vi "Nuevo Asistente.vi"(8 "error in (no error)":errorcluster) -> (0 "error out":errorcluster, 1 "Datos de Nueva Adquisición":T1={"Equipo a Utilizar"=enum."TDS 2012B Osciloscope", "Montura"=enum."Motor Bipolar", "Datos Zaber"={"Sentido de Adquisición"=FALSE, "Comenzar Desde Home?"=FALSE, "Distancia a recorrer (um)"=0.0, "Pasos motor"=0, "Distancia entre Lecturas (um)"=0.0, "Puerto"=""}, "Datos Bipolar/Unipolar"={"Puerto COM"="", "Pasos entre Lecturas"=0, "Numero de lecturas"=0, "Sentido del motor"=TRUE}, "Datos Archivo"={"Ruta Archivo"=path "", "Nombre de Prueba"=""}, "Datos actuales"={"Montura"="", "Equipo"="", "Posición Actual"="", "Distancia Total a recorrer"="", "distancia Entre lecturas"="", "Pasos entre lecturas"=""}, "Datos a Guardar In"={"Datos Cursor Tektronix"="", "Datos Lokin"="", "Posición Cero"=0.0, "Posición Actual"=0.0}, "Datos Osciloscopio"={"Sesión Visa Osciloscopio"="Tektronix_TDS2012C", "Tipo de Adquisición"=enum."Voltaje Pico Pico", "Canal a Utilizar"=enum."Canal 1", "Parametros de Adquisición"=enum."Una Muestra", "Número Promedio"=2}, "Datos Lock In"={"Visa Lock in"="Tektronix_TDS2012C"}} {"Datos Osciloscopio"."Número Promedio" min=2 max=20; "Datos a Guardar In"."Posición Actual" format="%#_10f"; "Datos a Guardar In"."Posición Cero" format="%#_10f"; "Datos Bipolar/Unipolar"."Numero de lecturas" max=910098 step=1}, 2 "Iniciar Prueba":bool)   [LabVIEW 2020]
doc: "Este VI es un asistente tipo \"wizzard\" para obtener los parámetros de una nueva prueba, captura el tipo de montura, cuantos pasos por lectura, equipo para lectura y ruta de almacenamiento de datos, nombre de la prueba."
uses:
  Type Definitions/tab wizard.ctl
  Type Definitions/Asistente de adquisicion Cluster.ctl
  Type Definitions/Datos a Guardar.ctl
  Type Definitions/datos osciloscopio.ctl
  Type Definitions/Datos Zaber.ctl
  Type Definitions/parametros motores.ctl
  <vilib>/Utility/sysdir.llb/System Directory Type.ctl
  H:/Mi unidad/Departamento de Ingenieria/Investigadores/Gabriel Ramos/Proyecto Monturas v13/LV Source/Type Definitions/Tipos de montura.ctl
panel:
  in  "Cancel Button":bool
  in  "Previous Button":bool
  in  "Next Button":bool
  out "Tab general":T7
  in  "Tipo de montura/Motor":T2
  in  "Datos Zaber":T3={"Sentido de Adquisición"=TRUE, "Comenzar Desde Home?"=TRUE, "Distancia a recorrer (um)"=2.0, "Pasos motor"=0, "Distancia entre Lecturas (um)"=0.1, "Puerto"="COM4"}
  in  "Datos Bipolar/Unipolar":T4 {"Numero de lecturas" max=910098 step=1}
  in  "Seleccion Equipo de medición":enum16{"SR830 Lock In", "TDS 2012B Osciloscope"}(ring)=enum."TDS 2012B Osciloscope"
  in  "Datos Osciloscopio":T6={"Sesión Visa Osciloscopio"="USB0::0x0699::0x0368::C017587::INSTR", "Tipo de Adquisición"=enum."Voltaje Pico Pico", "Canal a Utilizar"=enum."Canal 1", "Parametros de Adquisición"=enum."Una Muestra", "Número Promedio"=2} {"Número Promedio" min=2 max=20}
  in  "Puerto GPIB Lock In":refnum<visa-resource-name>="GPIB0::8::INSTR"
  in  "Datos Archivo":T8
  # "ENA"
  # "Bienvenido al Asistente de adquisición Automatizado\n\nEste asistente le ayudará a:\n\n* Seleccionar motor-montura a usar\n     -Zaber                  (USB-RS232C)\n     -Motor Unipolar     (COM Port)\n     -Motor Bipolar       (COM Port)\n\n* Seleccionar Instrumento de adquisición\n     -Lock-In Amplifier         SR830\n     -Osciloscopio               TDS-2012B\n\n* Parametros de adquisición\n    -Guardado de Archivo\n    -Pasos por lectura"
  # "Motor Unipolar"
  # "Motor Bipolar"
  # "Zaber"
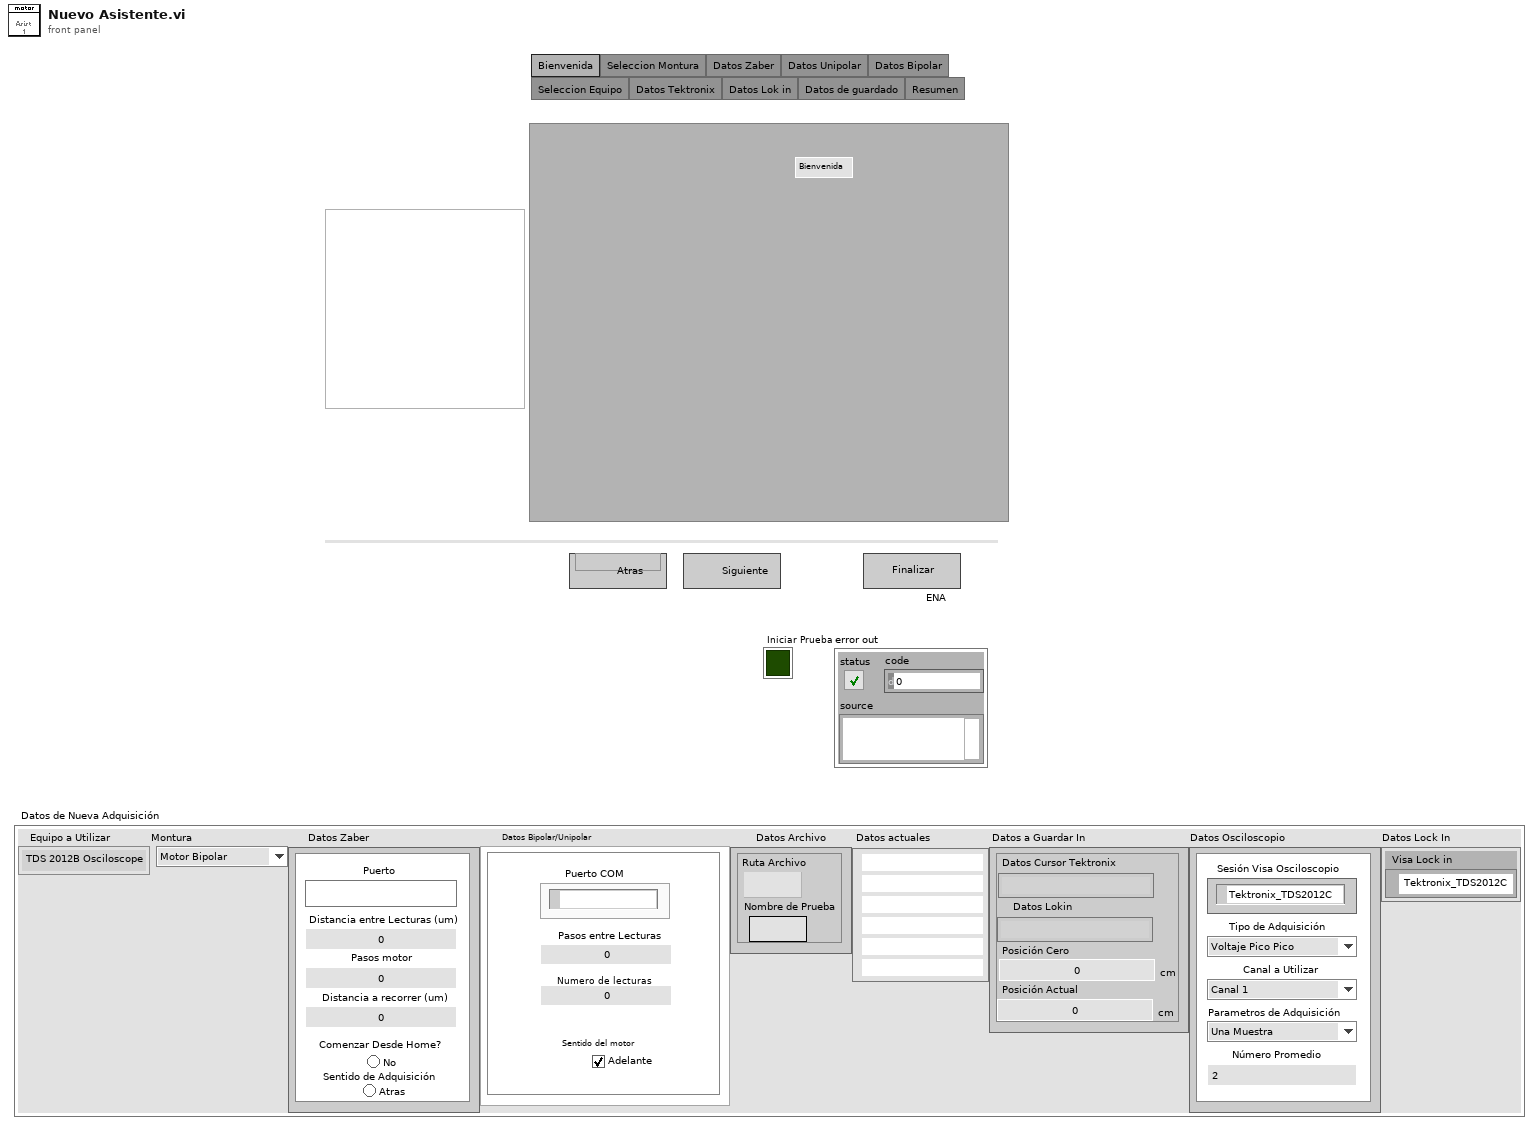
[diagram p1: front panel]
types:
  T1 = typedef "Asistente de adquisicion Cluster.ctl" = cluster{"Equipo a Utilizar":enum16{"SR830 Lock In", "TDS 2012B Osciloscope"}, "Montura":T2, "Datos Zaber":T3, "Datos Bipolar/Unipolar":T4, "Datos Archivo":cluster{"Ruta Archivo":path, "Nombre de Prueba":string}, "Datos actuales":cluster{"Montura":string, "Equipo":string, "Posición Actual":string, "Distancia Total a recorrer":string, "distancia Entre lecturas":string, "Pasos entre lecturas":string}, "Datos a Guardar In":T5, "Datos Osciloscopio":T6, "Datos Lock In":cluster{"Visa Lock in":refnum<visa-resource-name>}}
  T2 = typedef "Tipos de montura.ctl" = enum16{"Zaber T-LSR450B", "Zaber-T-LSR300B", "Zaber-T-LSRxxx", "Motor Bipolar", "Motor Unipolar"}
  T3 = typedef "Datos Zaber.ctl" = cluster{"Sentido de Adquisición":bool, "Comenzar Desde Home?":bool, "Distancia a recorrer (um)":dbl, "Pasos motor":i32, "Distancia entre Lecturas (um)":dbl, "Puerto":refnum<visa-resource-name>}
  T4 = typedef "parametros motores.ctl" = cluster{"Puerto COM":refnum<visa-resource-name>, "Pasos entre Lecturas":u16, "Numero de lecturas":u32, "Sentido del motor":bool}
  T5 = typedef "Datos a Guardar.ctl" = cluster{"Datos Cursor Tektronix":string, "Datos Lokin":string, "Posición Cero":dbl[unit], "Posición Actual":dbl[unit]}
  T6 = typedef "datos osciloscopio.ctl" = cluster{"Sesión Visa Osciloscopio":refnum<visa-resource-name>, "Tipo de Adquisición":enum16{"Voltaje Pico Pico", "Voltaje RMS", "Cursor Tiempo"}, "Canal a Utilizar":enum16{"Canal 1", "Canal 2", "Canal 1 y 2"}, "Parametros de Adquisición":enum16{"Una Muestra", "Promedio"}, "Número Promedio":i32}
  T7 = typedef "tab wizard.ctl" = enum32{"Bienvenida", "Seleccion Montura", "Datos Zaber", "Datos Unipolar", "Datos Bipolar", "Seleccion Equipo", "Datos Tektronix", "Datos Lok in", "Datos de guardado", "Resumen"}
  T8 = cluster{"Ruta Archivo":path, "Nombre de Prueba":string}
  T9 = typedef "System Directory Type.ctl" = i32
  T10 = enum8{"Enabled", "Disabled", "Disabled and Grayed Out"}
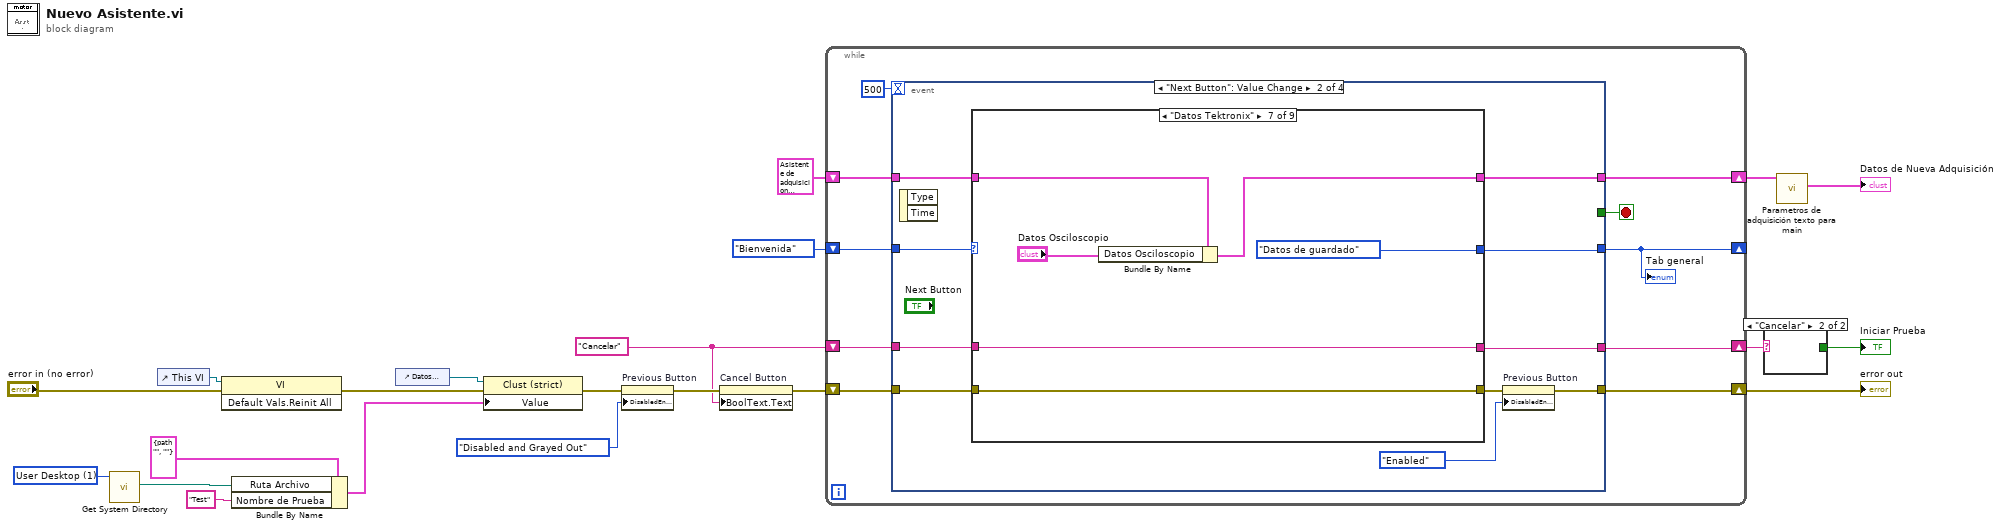
[diagram p0: block diagram]
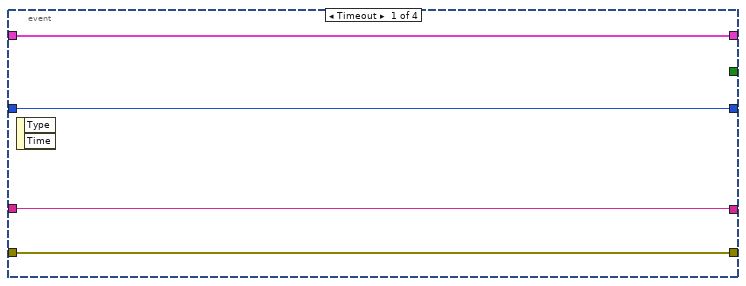
[diagram p2: hidden frame]
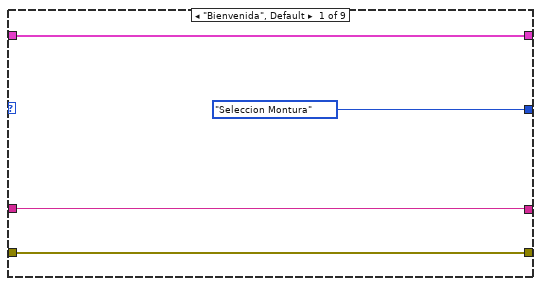
[diagram p3: hidden frame]
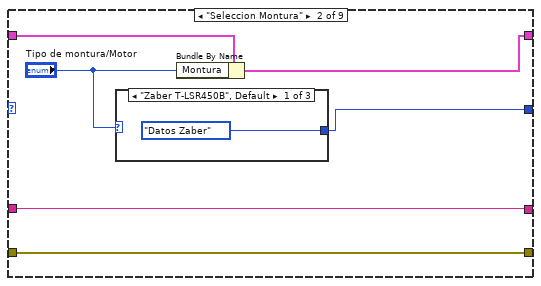
[diagram p4: hidden frame]
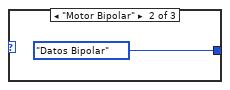
[diagram p5: hidden frame]
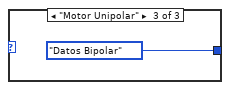
[diagram p6: hidden frame]
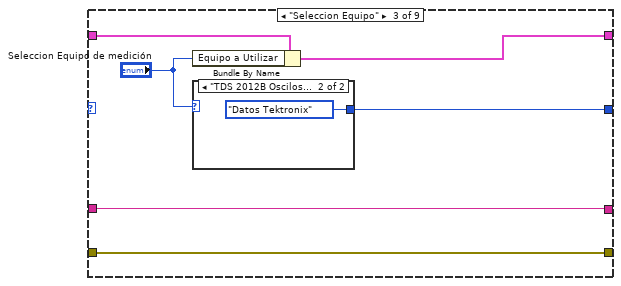
[diagram p7: hidden frame]
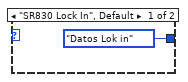
[diagram p8: hidden frame]
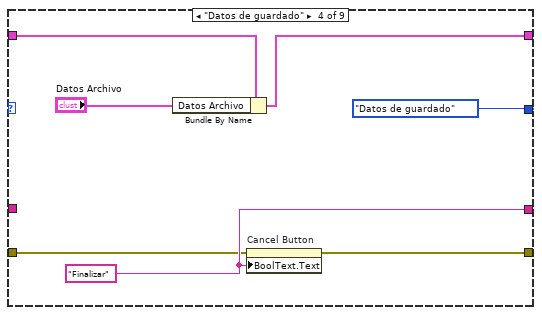
[diagram p9: hidden frame]
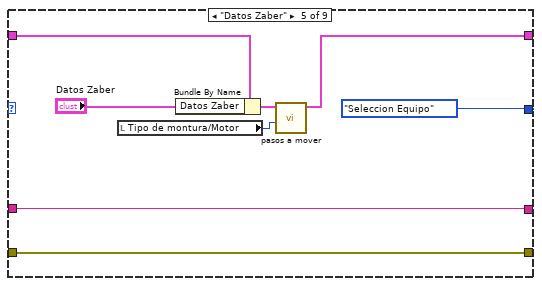
[diagram p10: hidden frame]
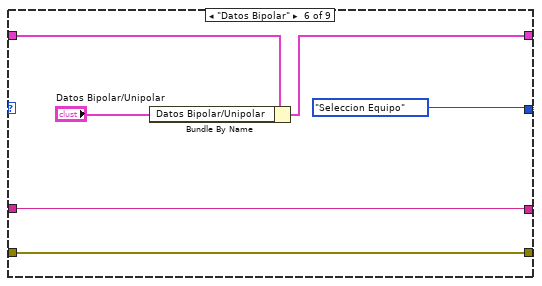
[diagram p11: hidden frame]
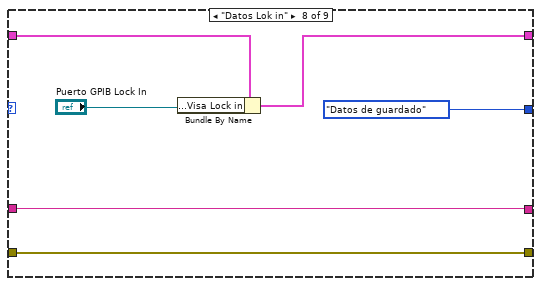
[diagram p12: hidden frame]
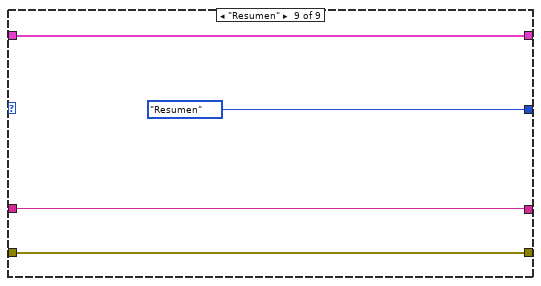
[diagram p13: hidden frame]
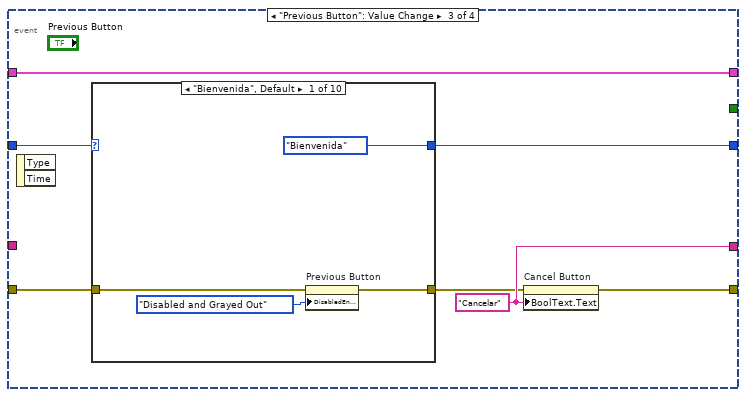
[diagram p14: hidden frame]
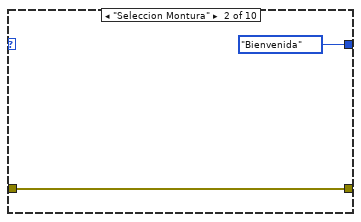
[diagram p15: hidden frame]
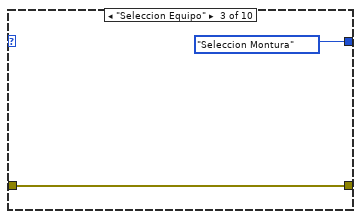
[diagram p16: hidden frame]
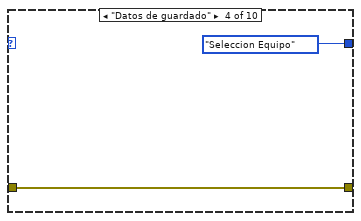
[diagram p17: hidden frame]
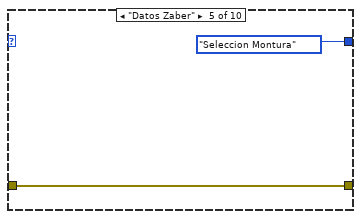
[diagram p18: hidden frame]
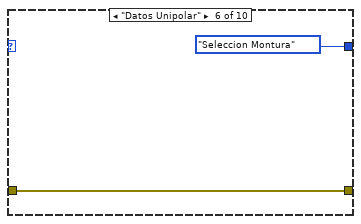
[diagram p19: hidden frame]
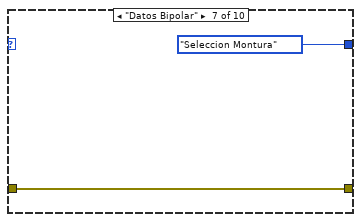
[diagram p20: hidden frame]
diagram:
  w11 = T9 1 items=["User Home"=0, "User Desktop"=1, "User Documents"=2, "User Application Data"=3, "User Preferences"=4, "User Temporary"=5, "Public Documents"=6, "Public Application Data"=7, "Public Preferences"=8, "Public Cache"=13, "System Core Libraries"=9, "System Installed Libraries"=10, "Application Files"=11, "Boot Volume Root"=12] ("system directory type")
  w16 = "Cancelar" ("Boolean Text.Text")
  n1 = call <vilib>:"Get System Directory.vi"("system directory type"=w11) -> ("system directory"=w12:path)  [unwired: 10 in]
  n2 = control-ref of="This VI"() -> (w7:refnum<vi>)
  n3 = invoke class="VI" method="Default Vals.Reinit All"(reference=w7, error in="error in (no error)") -> (error out=w2:errorcluster)  [unwired: 1 in, 2 out]
  n4 = Bundle By Name(cluster=T8 {"Ruta Archivo"=path "", "Nombre de Prueba"=""} ("Value"), "Ruta Archivo"=w12, "Nombre de Prueba"="Test") -> (w10:T8)
  n5 = control-ref of="Datos Archivo"() -> (w14:refnum<vi>)
  n6 = property class="Clust (strict)"(reference=w14, error in=w2, "Value"=w10) -> (error out=w8:errorcluster)  [unwired: 1 out]
  n7 = property on="Previous Button" class="Bool"(error in=w8, "DisabledEnum"=T10."Disabled and Grayed Out" ("Disabled")) -> (error out=w20:errorcluster)  [unwired: 1 in, 1 out]
  n8 = property on="Cancel Button" class="Bool"(error in=w20, "BoolText.Text"=w16) -> (error out=w3:errorcluster)  [unwired: 1 in, 1 out]
  n9 = while {
    shift-right: [w26] -> _
    shift-left: tab_wizard."Bienvenida" ("Tab general") -> [w29]
    shift-right: [w28] -> w19
    shift-left: w16 -> [w27]
    shift-right: [w24] -> w17
    shift-left: w3 -> [w25]
    shift-right: [w22] -> w5
    shift-left: T1 {"Equipo a Utilizar"=enum."TDS 2012B Osciloscope", "Montura"=enum."Motor Bipolar", "Datos Zaber"={"Sentido de Adquisición"=FALSE, "Comenzar Desde Home?"=FALSE, "Distancia a recorrer (um)"=0.0, "Pasos motor"=0, "Distancia entre Lecturas (um)"=0.0, "Puerto"=""}, "Datos Bipolar/Unipolar"={"Puerto COM"="", "Pasos entre Lecturas"=0, "Numero de lecturas"=0, "Sentido del motor"=TRUE}, "Datos Archivo"={"Ruta Archivo"=path "", "Nombre de Prueba"=""}, "Datos actuales"={"Montura"="", "Equipo"="", "Posición Actual"="", "Distancia Total a recorrer"="", "distancia Entre lecturas"="", "Pasos entre lecturas"=""}, "Datos a Guardar In"={"Datos Cursor Tektronix"="", "Datos Lokin"="", "Posición Cero"=0.0, "Posición Actual"=0.0}, "Datos Osciloscopio"={"Sesión Visa Osciloscopio"="Tektronix_TDS2012C", "Tipo de Adquisición"=enum."Voltaje Pico Pico", "Canal a Utilizar"=enum."Canal 1", "Parametros de Adquisición"=enum."Una Muestra", "Número Promedio"=2}, "Datos Lock In"={"Visa Lock in"="Tektronix_TDS2012C"}} ("Datos de Nueva Adquisición In") -> [w23]
    stop <- w30 stop-if-true
    n10 = event shown="[1] \"Next Button\": Value Change" {
      selector: _ -> [_ _ _ _]
      dyn-events: _ -> [_ _ _ _]
      timeout: 500 -> [_ _ _ _]
      tunnel: [_ _ _ "Cancel Button"] -> w30
      tunnel: w29 -> [w34 w41 w109 w135]
      tunnel: [w35 w44 w110 w136] -> w28
      tunnel: w27 -> [w35 w43 _ w136]
      tunnel: [w34 w42 w108 w135] -> w26
      tunnel: w25 -> [w33 w40 w105 w134]
      tunnel: [w33 w38 w107 w134] -> w24
      tunnel: w23 -> [w32 w37 w106 w133]
      tunnel: [w32 w36 w106 w133] -> w22
      event Timeout {
        n11 = event-data() -> ()  [unwired: 1 in, 2 out]
      }
      event "Next Button": Value Change {
        n12 = event-data() -> ()  [unwired: 1 in, 2 out]
        n13 = case shown="\"Datos Tektronix\"" w41 {
          tunnel: [w49 w54 w64 w73 w80 w85 w91 w97 w102] -> w44
          tunnel: w43 -> [w49 w54 w64 _ w80 w85 w91 w97 w102]
          tunnel: [tab_wizard."Seleccion Montura" ("Tab general") w55 w62 tab_wizard."Datos de guardado" ("Tab general") tab_wizard."Seleccion Equipo" ("Tab general") tab_wizard."Seleccion Equipo" ("Tab general") tab_wizard."Datos de guardado" ("Tab general") tab_wizard."Datos de guardado" ("Tab general") tab_wizard."Resumen" ("Tab general")] -> w42
          tunnel: w40 -> [w47 w53 w63 w71 w79 w86 w93 w98 w103]
          tunnel: [w47 w53 w63 w70 w79 w86 w93 w98 w103] -> w39
          tunnel: w37 -> [w46 w52 w61 w69 w78 w84 w90 w96 w101]
          tunnel: [w46 w51 w60 w67 w75 w83 w89 w95 w101] -> w36
          frame "Bienvenida", Default {
          }
          frame "Seleccion Montura" {
            n14 = case shown="\"Zaber T-LSR450B\", Default" "Tipo de montura/Motor" {
              tunnel: [tab_wizard."Datos Zaber" ("Tab general") tab_wizard."Datos Bipolar" ("Tab general") tab_wizard."Datos Bipolar" ("Tab general")] -> w55
              frame "Zaber T-LSR450B", Default {
              }
              frame "Motor Bipolar" {
              }
              frame "Motor Unipolar" {
              }
            }
            n15 = Bundle By Name(cluster=w52, "Montura"="Tipo de montura/Motor") -> (w51:T1)
          }
          frame "Seleccion Equipo" {
            n16 = Bundle By Name(cluster=w61, "Equipo a Utilizar"="Seleccion Equipo de medición") -> (w60:T1)
            n17 = case shown="\"TDS 2012B Osciloscope\"" "Seleccion Equipo de medición" {
              tunnel: [tab_wizard."Datos Lok in" ("Tab general") tab_wizard."Datos Tektronix" ("Tab general")] -> w62
              frame "SR830 Lock In", Default {
              }
              frame "TDS 2012B Osciloscope" {
              }
            }
          }
          frame "Datos de guardado" {
            w73 = "Finalizar" ("Boolean Text.Text")
            n18 = Bundle By Name(cluster=w69, "Datos Archivo"="Datos Archivo") -> (w67:T1)
            n19 = property on="Cancel Button" class="Bool"(error in=w71, "BoolText.Text"=w73) -> (error out=w70:errorcluster)  [unwired: 1 in, 1 out]
          }
          frame "Datos Zaber" {
            n20 = local read "Tipo de montura/Motor"() -> (w74:T2)
            n21 = Bundle By Name(cluster=w78, "Datos Zaber"="Datos Zaber") -> (w76:T1)
            n22 = call "pasos a mover.vi"("Montura"=w74, "Datos de Nueva Adquisición In"=w76) -> ("Datos nueva adquisición Out"=w75:T1)  [unwired: 9 in]
          }
          frame "Datos Bipolar" {
            n23 = Bundle By Name(cluster=w84, "Datos Bipolar/Unipolar"="Datos Bipolar/Unipolar") -> (w83:T1)
          }
          frame "Datos Tektronix" {
            n24 = Bundle By Name(cluster=w90, "Datos Osciloscopio"="Datos Osciloscopio") -> (w89:T1)
          }
          frame "Datos Lok in" {
            n25 = Bundle By Name(cluster=w96, "Datos Lock In.Visa Lock in"="Puerto GPIB Lock In") -> (w95:T1)
          }
          frame "Resumen" {
          }
        }
        n26 = property on="Previous Button" class="Bool"(error in=w39, "DisabledEnum"=T10."Enabled" ("Disabled")) -> (error out=w38:errorcluster)  [unwired: 1 in, 1 out]
      }
      event "Previous Button": Value Change {
        w110 = "Cancelar" ("Boolean Text.Text")
        n27 = event-data() -> ()  [unwired: 1 in, 2 out]
        n28 = case shown="\"Bienvenida\", Default" w109 {
          tunnel: [tab_wizard."Bienvenida" ("Tab general") tab_wizard."Bienvenida" ("Tab general") tab_wizard."Seleccion Montura" ("Tab general") tab_wizard."Seleccion Equipo" ("Tab general") tab_wizard."Seleccion Montura" ("Tab general") tab_wizard."Seleccion Montura" ("Tab general") tab_wizard."Seleccion Montura" ("Tab general") tab_wizard."Seleccion Equipo" ("Tab general") tab_wizard."Seleccion Equipo" ("Tab general") tab_wizard."Seleccion Equipo" ("Tab general")] -> w108
          tunnel: w105 -> [w112 w115 w117 w119 w122 w124 w125 w127 w129 w132]
          tunnel: [w111 w115 w117 w119 w122 w124 w125 w127 w129 w132] -> w104
          frame "Bienvenida", Default {
            n29 = property on="Previous Button" class="Bool"(error in=w112, "DisabledEnum"=T10."Disabled and Grayed Out" ("Disabled")) -> (error out=w111:errorcluster)  [unwired: 1 in, 1 out]
          }
          frame "Seleccion Montura" {
          }
          frame "Seleccion Equipo" {
          }
          frame "Datos de guardado" {
          }
          frame "Datos Zaber" {
          }
          frame "Datos Unipolar" {
          }
          frame "Datos Bipolar" {
          }
          frame "Datos Tektronix" {
          }
          frame "Datos Lok in" {
          }
          frame "Resumen" {
          }
        }
        n30 = property on="Cancel Button" class="Bool"(error in=w104, "BoolText.Text"=w110) -> (error out=w107:errorcluster)  [unwired: 1 in, 1 out]
      }
      event "Cancel Button": Value Change {
        n31 = event-data() -> ()  [unwired: 1 in, 2 out]
      }
    }
    "Tab general" <- w26
  }
  "error out" <- w17
  n32 = case shown="\"Cancelar\"" w19 {
    tunnel: [TRUE _] -> w18
    frame "Finalizar", Default {
    }
    frame "Cancelar" {
    }
  }
  "Iniciar Prueba" <- w18
  n33 = call "Parametros de adquisición texto para main.vi"("Datos de Nueva Adquisición in"=w5) -> ("Datos de Nueva Adquisición out"=→"Datos de Nueva Adquisición":T1)  [unwired: 10 in]
